vi "3.1.12-Detect Lidar Setpoint.vi"(0 "Enum 2":T3(ring), 1 "Ref Out":T1, 2 "User want to get on with his life":bool, 5 "Has Refrence":bool) -> (3 "Lidar Motor Position Integer @ Home":i32, 4 "Enum":T3(ring), 6 "Waveform Chart":dbl[](graph), 7 "Positive Inflexion Point":bool, 8 "2.1 Act Debug":T2, 9 "FPGA VI Reference Out":T1, 10 "Lidar Position Integer @ Home":i32)   [LabVIEW 2010]
uses:
  2-Low Neurons/2.1 Act Debug.ctl
  2-Low Neurons/2-FPGA VI Typedef.ctl
  <vilib>/rvi/interface/nirviReadWriteControl/nirviReadWriteControl.xnode
  FPGA Bitfiles/DaveBrain_FPGATarget_1-Hindbrain_F0E489D8.lvbitx
  1-Hindbrain.vi
  <vilib>/rvi/interface/common/niFpgaNodeNameForErrorReporting.ctl
  <vilib>/rvi/errors/niLvFpgaWhatHappensToTopLevelVI.ctl
  <vilib>/RVI Host/nirviSupport.llb/nirviErrorClusterFromErrorCode.vi
  <vilib>/rvi/errors/niLvFpgaAdjustHostInterfaceError.vi
  3.0-Global.vi
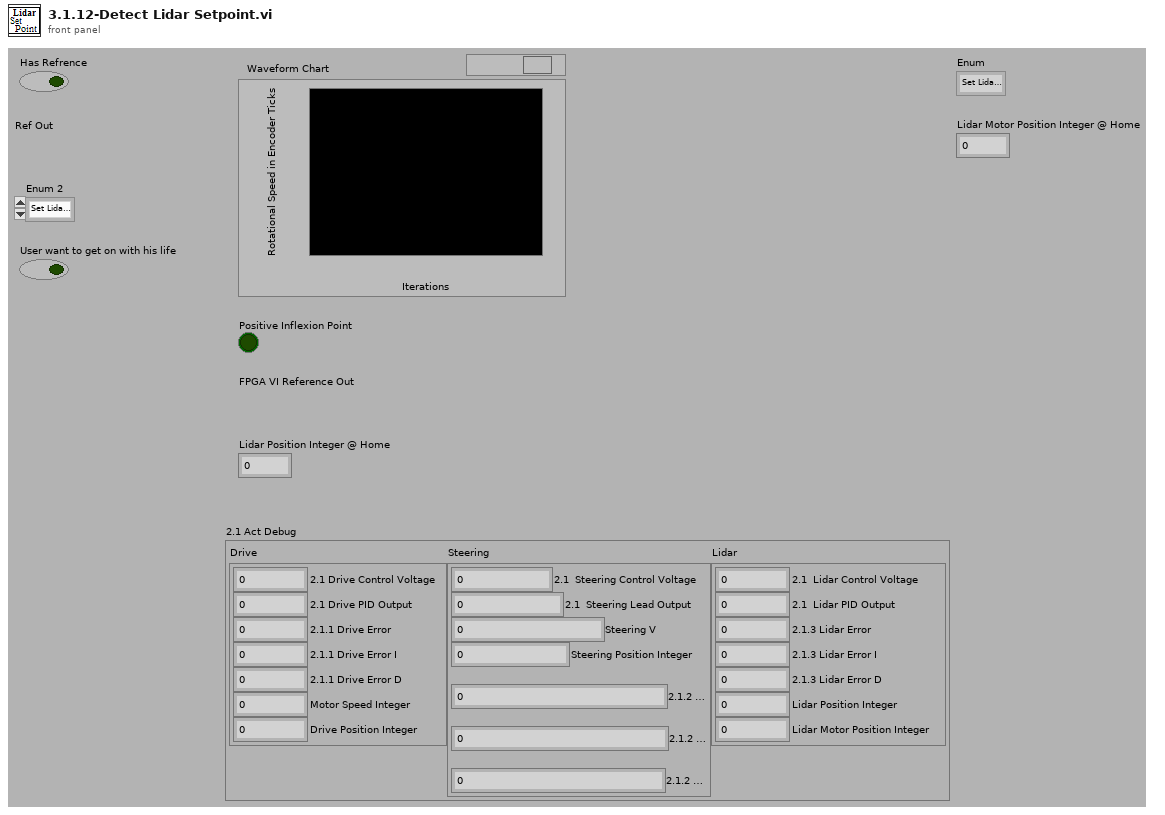
[diagram p1: front panel]
types:
  T1 = typedef "2-FPGA VI Typedef.ctl" = refnum<k20>
  T2 = typedef "2.1 Act Debug.ctl" = cluster{"Drive":cluster{"2.1 Drive Control Voltage":fxp<+/-,20,5>, "2.1 Drive PID Output":fxp<+/-,20,5>, "2.1.1 Drive Error":fxp<+/-,18,1>, "2.1.1 Drive Error I":fxp<+/-,64,46>, "2.1.1 Drive Error D":fxp<+/-,18,1>, "Motor Speed Integer":fxp<+/-,10,8>, "Drive Position Integer":i32}, "Steering":cluster{"2.1  Steering Control Voltage":fxp<+/-,20,5>, "2.1  Steering Lead Output":fxp<+/-,20,5>, "Steering V":fxp<+/-,10,8>, "Steering Position Integer":i32, "2.1.2 sqrt(10)s+bdt":fxp<+/-,18,20>, "2.1.2 (sqrt(10)s+bdt)/(s/sqrt(10)+bdt)":fxp<+/-,20,22>, "2.1.2 s(sqrt(10)s+bdt)/(s/sqrt(10)+bdt)":fxp<+/-,20,22>}, "Lidar":cluster{"2.1  Lidar Control Voltage":fxp<+/-,20,5>, "2.1  Lidar PID Output":fxp<+/-,20,5>, "2.1.3 Lidar Error":fxp<+/-,18,1>, "2.1.3 Lidar Error I":fxp<+/-,64,46>, "2.1.3 Lidar Error D":fxp<+/-,18,1>, "Lidar Position Integer":i32, "Lidar Motor Position Integer":i32}}
  T3 = enum16{"Set Lidar Rotation", "Wait for Lidar Crossover Point", "Stop Lidar, Set Global", "Set Tentative Steering Zero", "Move Setpoint Left", "Move Setpoint Right", "Re-Calibrate Steering Zero"}
  T4 = typedef "niFpgaNodeNameForErrorReporting.ctl" = enum16{"Open FPGA VI Reference", "Read/Write Control", "Invoke Method: Abort", "Invoke Method: Acknowledge IRQ", "Invoke Method: Download", "Invoke Method: FIFO.Configure", "Invoke Method: FIFO.Read", "Invoke Method: FIFO.Start", "Invoke Method: FIFO.Stop", "Invoke Method: FIFO.Write", "Invoke Method: Reset", "Invoke Method: Run", "Invoke Method: Wait on IRQ", "Close FPGA VI Reference"}
  T5 = typedef "niLvFpgaWhatHappensToTopLevelVI.ctl" = enum16{"top level VI scripted behind XNode", "top level VI inlined behind XNode"}
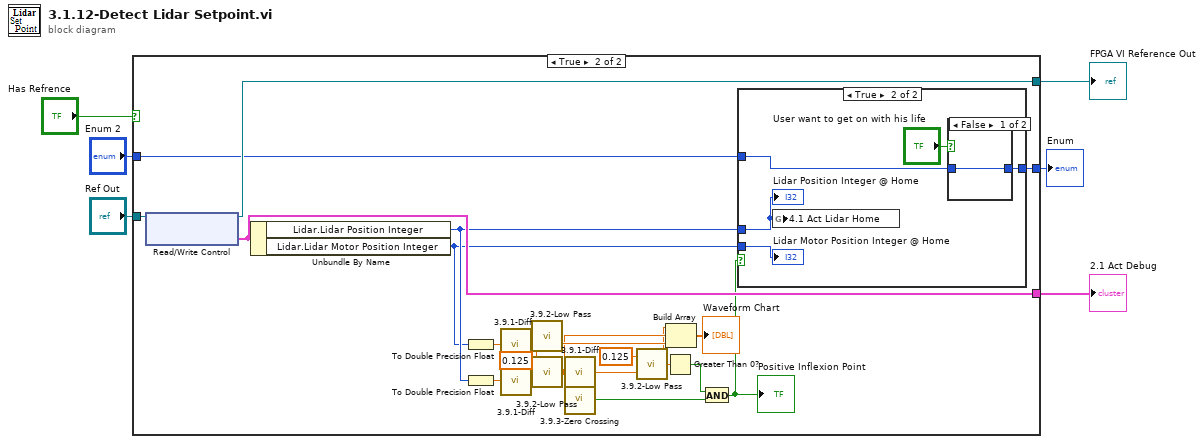
[diagram p0: block diagram]
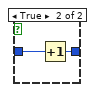
[diagram p4: hidden frame]
diagram:
  n1 = case shown="True" "Has Refrence" {
    tunnel: "Ref Out" -> [w8 w29]
    tunnel: [w8 w28] -> w1
    tunnel: [_ w25] -> w4
    tunnel: "Enum 2" -> [w7 w27]
    tunnel: [w7 w26] -> w6
    frame False {
    }
    frame True {
      w20 = 0.125 ("Low pass")
      n2 = xnode "Read/Write Control"("FPGA VI Reference In"=w29) -> ("FPGA VI Reference Out"=w28:T1, "2.1 Act Debug"=w25:T2)  [unwired: 1 in, 1 out]
      n3 = Unbundle By Name(w25) -> ("Lidar.Lidar Position Integer"=w10:i32, "Lidar.Lidar Motor Position Integer"=w9:i32)
      n4 = To Double Precision Float(number=w9) -> (double precision float=w23:dbl)
      n5 = To Double Precision Float(number=w10) -> (double precision float=w24:dbl)
      n6 = call "3.9.1-Diff.vi"("Numeric"=w23) -> ("Numeric 2"=w21:dbl)
      n7 = call "3.9.1-Diff.vi"("Numeric"=w24) -> ("Numeric 2"=w22:dbl)
      n8 = call "3.9.2-Low Pass.vi"("Signal In"=w21, "Gain"=w20) -> ("Signal Out"=w16:dbl)
      n9 = call "3.9.2-Low Pass.vi"("Signal In"=w22, "Gain"=w20) -> ("Signal Out"=w15:dbl)
      n10 = call "3.9.1-Diff.vi"("Numeric"=w15) -> ("Numeric 2"=w19:dbl)
      n11 = call "3.9.3-Zero Crossing.vi"("Signal Out"=w15) -> ("Boolean"=w12:bool)
      n12 = call "3.9.2-Low Pass.vi"("Signal In"=w19, "Gain"=0.125 ("Low pass")) -> ("Signal Out"=w14:dbl)
      n13 = Greater Than 0?(x=w14) -> (x > 0?=w13:bool)
      n14 = Build Array(w14, w15, w16) -> (→"Waveform Chart":dbl[])
      n15 = And(x=w13, y=w12) -> (x .and. y?=w11:bool)
      "Positive Inflexion Point" <- w11
      n16 = case shown="True" w11 {
        tunnel: w27 -> [w30 w35]
        tunnel: [w30 w34] -> w26
        tunnel: w10 -> [_ w32]
        tunnel: w9 -> [_ w33]
        frame False {
        }
        frame True {
          n17 = global write "3.0-Global.vi" "4.1 Act Lidar Home"(w32) -> ()
          n18 = case shown="False" "User want to get on with his life" {
            tunnel: w35 -> [w36 w38]
            tunnel: [w36 w37] -> w34
            frame False {
            }
            frame True {
              n19 = Increment(x=w38) -> (x+1=w37:T3)
            }
          }
          "Lidar Motor Position Integer @ Home" <- w33
          "Lidar Position Integer @ Home" <- w32
        }
      }
    }
  }
  "Enum" <- w6
  "2.1 Act Debug" <- w4
  "FPGA VI Reference Out" <- w1
